vi "Voltage Sweep 2 Timed Struct.vi"(11 "Voltage Sweep Settings":T1={"Voltage Step (V)"=20.0, "Voltage Range (V)"={200, 400}, "Time Step (s)"=0.0, "Voltage Step Direction"=enum."High 2 Low"} {"Voltage Range (V)" scale=0.0..500.0}) -> (1 "Vector":dbl[](array[numeric]), 2 "V0":dbl, 3 "dT":i32)   [LabVIEW 2011]
uses:
  Controls/PID Voltage Seep Settings.ctl
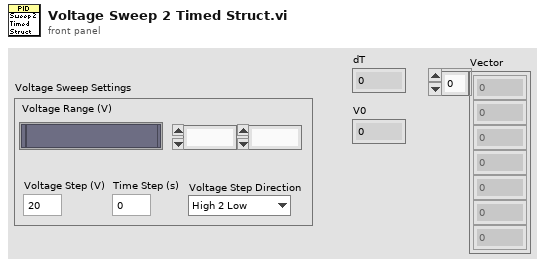
[diagram p1: front panel]
types:
  T1 = typedef "PID Voltage Seep Settings.ctl" = cluster{"Voltage Step (V)":dbl, "Voltage Range (V)":cluster{u16, u16}, "Time Step (s)":dbl, "Voltage Step Direction":enum16{"High 2 Low", "Low 2 High"}}
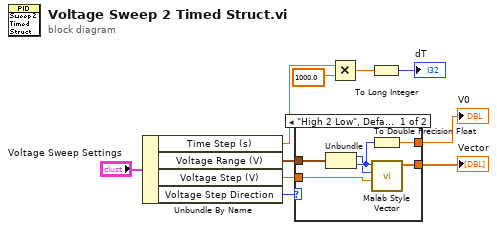
[diagram p0: block diagram]
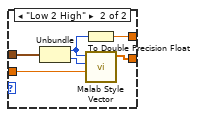
[diagram p2: hidden frame]
diagram:
  n1 = Unbundle By Name("Voltage Sweep Settings") -> ("Time Step (s)"=w7:dbl, "Voltage Range (V)"=w5:cluster{u16, u16}, "Voltage Step (V)"=w2:dbl, "Voltage Step Direction"=w4:enum16{"High 2 Low", "Low 2 High"})
  n2 = case shown="\"High 2 Low\", Default" w4 {
    tunnel: w5 -> [w16 w22]
    tunnel: [w15 w21] -> w3
    tunnel: w2 -> [w12 w18]
    tunnel: [w11 w17] -> w1
    frame "High 2 Low", Default {
      n3 = Unbundle(w16) -> (w13:u16, w14:u16)
      n4 = To Double Precision Float(number=w14) -> (double precision float=w15:dbl)
      n5 = call "Malab Style Vector.vi"("dt"=w12, "b"=w13, "a"=w14) -> ("Vector"=w11:dbl[])  [unwired: 8 in]
    }
    frame "Low 2 High" {
      n6 = Unbundle(w22) -> (w20:u16, w19:u16)
      n7 = To Double Precision Float(number=w20) -> (double precision float=w21:dbl)
      n8 = call "Malab Style Vector.vi"("dt"=w18, "b"=w19, "a"=w20) -> ("Vector"=w17:dbl[])  [unwired: 8 in]
    }
  }
  "V0" <- w3
  "Vector" <- w1
  n9 = Multiply(x=w7, y=1000.0) -> (x*y=w10:dbl)
  n10 = To Long Integer(number=w10) -> (32bit integer=→"dT":i32)
